vi "Get Size of Data from TD - Variant With Nested Variant Attributes - Returns Correct Size.vi"() -> ()   [LabVIEW 2017, in "Composition.Tests.lvlib"]
uses:
  Composition.Tests.lvlib
  <vilib>/addons/_JKI Toolkits/Caraya/classes/Assert/Assert Equal Value_Variant.vi
  Composition/Composition.lvlib
  <vilib>/addons/_JKI Toolkits/Caraya/classes/Test/Test.lvclass
  <vilib>/addons/_JKI Toolkits/Caraya/classes/Assert/Assert.lvclass
panel:
  out "error out":errorcluster
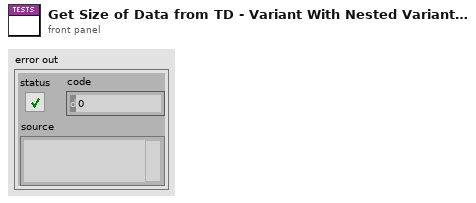
[diagram p1: front panel]
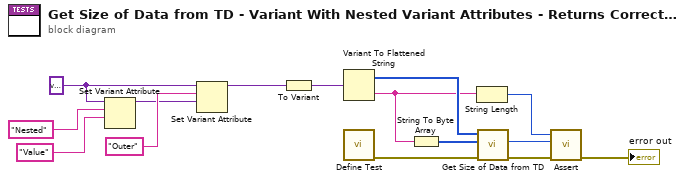
[diagram p0: block diagram]
diagram:
  w2 = variant
  n1 = Set Variant Attribute(Variant=w2, name="Nested", value="Value") -> (Variant out=w3:variant)  [unwired: 1 in, 2 out]
  n2 = Set Variant Attribute(Variant=w2, name="Outer", value=w3) -> (Variant out=w5:variant)  [unwired: 1 in, 2 out]
  n3 = To Variant(anything=w5) -> (Variant=w14:variant)
  n4 = Variant To Flattened String(Variant=w14) -> (data string=w7:string, 1:w8:i16[])
  n5 = call <vilib>:"Define Test.vi"() -> ("error out"=w13:errorcluster)  [unwired: 10 in, 1 out]
  n6 = String To Byte Array(string=w7) -> (unsigned byte array=w15:u8[])
  n7 = String Length(string=w7) -> (length=w9:i32)
  n8 = call "Get Size of Data from TD.vi"("error in (no error)"=w13, "Data String"=w15, "Type Descriptor"=w8) -> ("error out"=w12:errorcluster, "Size of Data"=w11:i32)  [unwired: 7 in]
  n9 = call-poly <vilib>:"Assert.vi"("error in (no error)"=w12, "Y"=w11, "X"=w9) -> ("error out"=→"error out":errorcluster)  [unwired: 7 in, 1 out]
